vi "Send Add Service.vi"(5 "Receive Connection Enqueuer Handler":refnum<class "WebSocket Server-Service Enqueuer Msg.lvclass">, 6 "WebSocket Data Handler":refnum<class "WebSocket Connection Handler Msg.lvclass">, 7 "Priority":T1=enum."Normal" caption="Message Priority (Normal)", 8 "error in (no error)":errorcluster, 9 "Subscriber Enqueuer":refnum<class "Message Enqueuer.lvclass">, 10 "Service Name":string, 11 "Message Enqueuer in":refnum<class "Message Enqueuer.lvclass">) -> (0 "error out":errorcluster, 3 "Message Enqueuer out":refnum<class "Message Enqueuer.lvclass">)   [LabVIEW 2021, in "WebSocket Actors.lvlib" / "Add Service Msg.lvclass"]
doc: "Sends the <b>WebSocket Actors.lvlib:Add Service Msg.lvclass</b> message.\n\nThis message will call <b>Add Service.vi</b> on the <b>WebSocket Actors.lvlib:WebSocket Server.lvclass</b> actor.\n\n<b>Add Service.vi Description</b>\nThis method will start a WebSocket service as specified by \"Service Name\". If the service is already running its enqueuer is returned to the subscriber, otherwise the service is also started, and the enqueuer returned."
uses:
  Add Service Msg.lvclass
  Add Service Msg.lvclass/Add Service Msg.ctl
  <vilib>/ActorFramework/Message Enqueuer/Message Enqueuer.lvclass
  C:/Program Files/National Instruments/LabVIEW 2021/vi.lib/ActorFramework/Message/Message.lvclass
  C:/Projects/Shared Libraries/WebSocket Actor/WebSocket Actor/WebSocket Server Messages/Add Service Msg/Add Service Msg.lvclass
  <vilib>/ActorFramework/Message Enqueuer/Message Priority.ctl
  Abstract Messages/WebSocket Server-Service Enqueuer Msg/WebSocket Server-Service Enqueuer Msg.lvclass
  Abstract Messages/WebSocket Connection Handler Msg/WebSocket Connection Handler Msg.lvclass
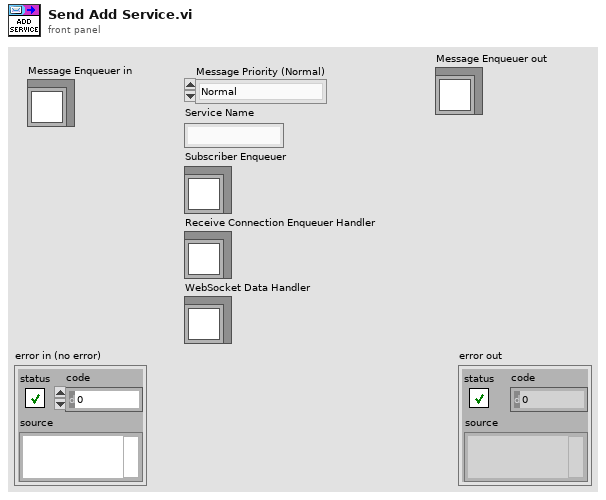
[diagram p1: front panel]
types:
  T1 = typedef "Actor Framework.lvlib/Message Enqueuer.lvclass/Message Priority.ctl" = enum16{"Low", "Normal", "High"}
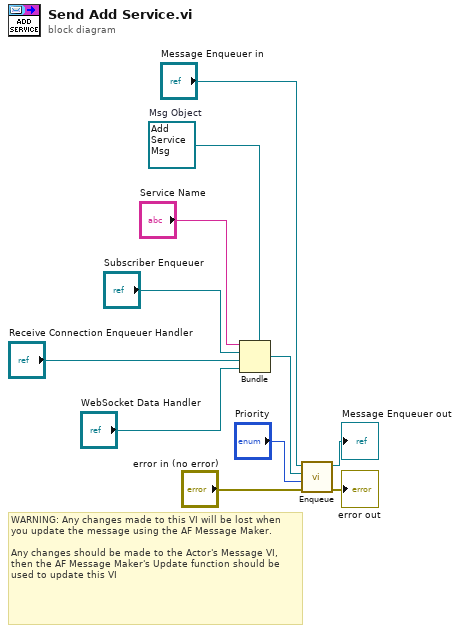
[diagram p0: block diagram]
diagram:
  w7 = refnum<class "Add Service Msg.lvclass"> refnum  # Msg Object
  # "WARNING: Any changes made to this VI will be lost when you update the message using the AF Message Maker.\n\nAny changes should be made to the Actor's Message VI, then the AF Message Maker's Update function should be used to update this VI"
  n1 = Bundle(cluster=w7, "Service Name", "Subscriber Enqueuer", "Receive Connection Enqueuer Handler", "WebSocket Data Handler") -> (w2:refnum<class "Add Service Msg.lvclass">)
  n2 = call <vilib>:"Enqueue.vi"("error in (no error)"="error in (no error)", "Message Priority (Normal)"="Priority", "Message"=w2, "Message Enqueuer in"="Message Enqueuer in") -> ("error out"=→"error out":errorcluster, "Message Enqueuer out"=→"Message Enqueuer out":refnum<class "Message Enqueuer.lvclass">)  [unwired: 6 in]
